vi "TransmitData.vi"(0 "设备类型":u32(ring)=3 items=["PCI5121"=1, "PCI9810"=2, "USBCAN1"=3, "USBCAN2"=4, "PCI9820"=5, "PCI5110"=7, "PC104CAN"=11, "CANETUDP"=12, "PCI9840B"=14, "PC104C2"=15, "PCI9820I"=16, "CANETTCP"=17, "PCIE9221"=24], 1 "帧类型":u8(ring) items=["标准帧", "扩展帧"], 2 "DeviceInd":u32, 5 "数据输入":string, 7 "ID":u32=1824 format="%08x", 9 "发送类型":u8(ring) items=["正常发送", "单次发送", "自发自收", "单次自发自收"], 11 "错误输入":errorcluster caption="错误输入（无错误）", 12 "帧格式":u8(ring) items=["数据帧", "远程帧"], 13 "CANInd":u32) -> (4 "DeviceType":u32, 6 "return type":u32, 8 "Result":bool, 10 "VCI_CAN_OBJT":T1 {"?" format="%.0x"}, 15 "错误输出":errorcluster)   [LabVIEW 2013]
uses:
  ControlCAN.dll
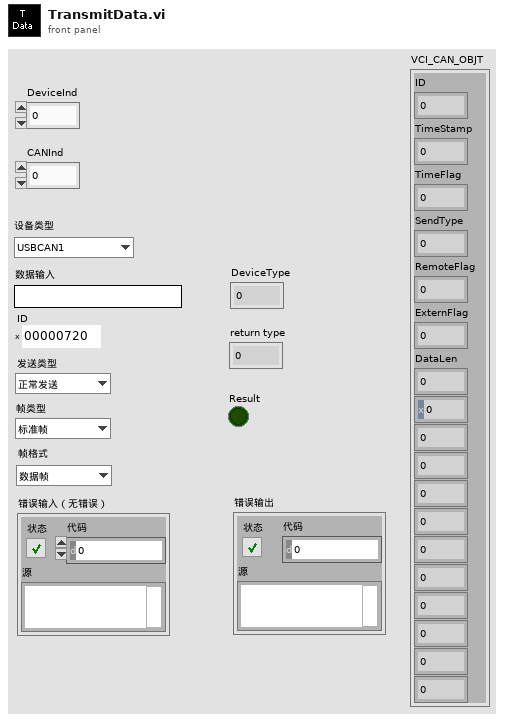
[diagram p1: front panel]
types:
  T1 = cluster{"ID":u32, "TimeStamp":u32, "TimeFlag":u8, "SendType":u8, "RemoteFlag":u8, "ExternFlag":u8, "DataLen":u8, u8, u8, u8, u8, u8, u8, u8, u8, u8, u8, u8}
  T2 = cluster{"[0]":u32, "[1]":u32, "[2]":u32, "[3]":u32, "[4]":u32, "[5]":u32, "[6]":u32, "[7]":u32, "[8]":u32}
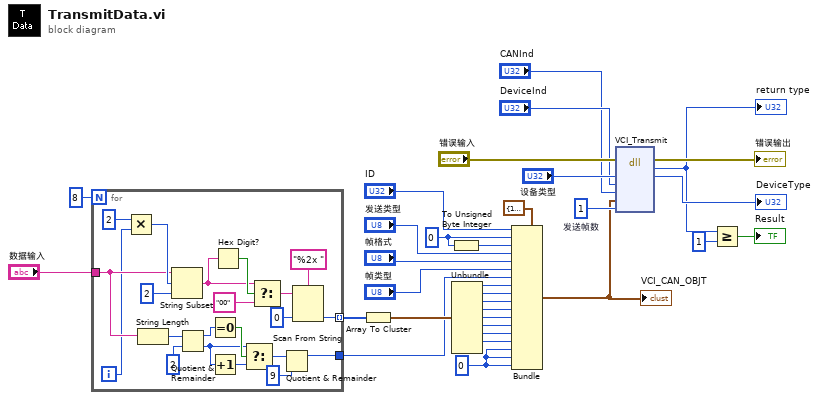
[diagram p0: block diagram]
diagram:
  w12 = u32 1  # 发送帧数
  w31 = u8 0
  w19 = u32 0
  n1 = for {
    N: 8 -> [_]
    tunnel: "数据输入" -> [w46]
    tunnel: [w49] -> w17 mode=indexing
    tunnel: [w34] -> w15
    i -> [w39]
    n2 = Multiply(x=2, y=w39) -> (x*y=w52:i32)
    n3 = String Length(string=w46) -> (length=w45:i32)
    n4 = String Subset(string=w46, offset (0)=w52, length (rest)=2 ("length (rest)")) -> (substring=w43:string)
    n5 = Quotient & Remainder(x=w45, y=2) -> (x-y*floor(x/y)=w41:i32, floor(x/y)=w37:i32)
    n6 = Equal To 0?(x=w41) -> (x = 0?=w40:bool)
    n7 = Increment(x=w37) -> (x+1=w38:i32)
    n8 = Hex Digit?(1:w43) -> (0:w47:bool)
    n9 = Select(t=w37, s=w40, f=w38) -> (s? t:f=w36:i32)
    n10 = Select(t=w43, s=w47, f="00" ("t")) -> (s? t:f=w48:string)
    n11 = Quotient & Remainder(x=w36, y=9) -> (x-y*floor(x/y)=w34:i32)  [unwired: 1 out]
    n12 = Scan From String(format string="%2x ", input string=w48, default 1=u32 0 ("默认值 1")) -> (output 1=w49:u32)  [unwired: 2 in, 3 out]
  }
  n13 = Array To Cluster(array=w17) -> (cluster=w16:T2)
  n14 = To Unsigned Byte Integer(number=w19) -> (unsigned 8bit integer=w18:u8)
  n15 = Unbundle(w16) -> ("[0]"=w23:u32, "[1]"=w24:u32, "[2]"=w25:u32, "[3]"=w26:u32, "[4]"=w27:u32, "[5]"=w28:u32, "[6]"=w29:u32, "[7]"=w30:u32)  [unwired: 1 out]
  n16 = Bundle(cluster=T1 {"ID"=1824, "TimeStamp"=0, "TimeFlag"=0, "SendType"=0, "RemoteFlag"=0, "ExternFlag"=0, "DataLen"=8, 3, 34, 241, 240, 0, 0, 0, 0, 0, 0, 0} ("VCI_CAN_OBJ_T"), "ID"="ID", "TimeStamp"=w19, "TimeFlag"=w18, "SendType"="发送类型", "RemoteFlag"="帧格式", "ExternFlag"="帧类型", "DataLen"=w15, w23, w24, w25, w26, w27, w28, w29, w30, w31, w31, w31) -> (w3:T1)
  "VCI_CAN_OBJT" <- w3
  n17 = dll-call lib="PTH1`abs E桌面休眠电流方案休眠电流源码20181130\nInstrumentCANControlCAN.dll" fn="VCI_Transmit"(error in="错误输入", "DeviceType"="设备类型", "DeviceInd"="DeviceInd", "CANInd"="CANInd", "pSend"=w3, "Len"=w12) -> (error out=→"错误输出":errorcluster, "return type"=w8:u32, "DeviceType"=→"DeviceType":u32)  [unwired: 5 in, 2 out]
  "return type" <- w8
  n18 = Greater Or Equal?(x=w8, y=u32 1) -> (x >= y?=→"Result":bool)
